vi "Generate Data Frame Vectors.vi"(0 "RFFE Command in":refnum<class "RFFE Command.lvclass">, 11 "error in (no error)":errorcluster) -> (4 "RFFE Command out":refnum<class "RFFE Command.lvclass">, 6 "Data Frame Vectors":string[](array[string]), 15 "error out":errorcluster)   [LabVIEW 2018, in "MIPI RFFE API.lvlib" / "RFFE Command.lvclass"]
uses:
  RFFE Command.lvclass
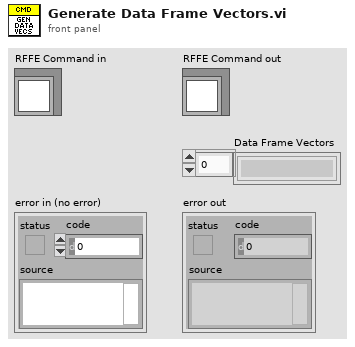
[diagram p1: front panel]
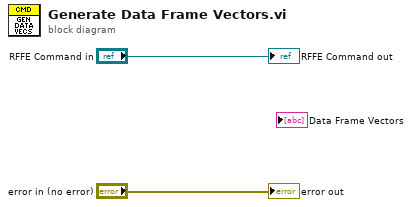
[diagram p0: block diagram]
diagram:
  "error out" <- "error in (no error)"
  "RFFE Command out" <- "RFFE Command in"
